vi "Update Plugin Status.vi"(6 "channels":T1, 8 "error in (no error)":errorcluster, 9 "Status":T5, 10 "Plugin Name":string, 11 "Launcher in":refnum<class "CIFPluginManager.lvclass">) -> (0 "error out":errorcluster)   [LabVIEW 2021, in "CIFPluginManager.lvclass"]
uses:
  CIFPluginManager.lvclass
  CIFPluginManager.lvclass/CIFPluginManager.ctl
  <vilib>/Utility/miscctls.llb/LVMapReplaceAction.ctl
  gRPC/CIF_Manager_server/RPC Messages/cif_management_common_PluginStatusData.ctl
  gRPC/CIF_Manager_server/CIF_Manager_server.lvlib
  gRPC/CIF_Manager_server/RPC Messages/cif_common_TimingStats.ctl
  gRPC/CIF_Manager_server/RPC Messages/cif_management_common_Channels.ctl
  gRPC/CIF_Manager_server/RPC Messages/cif_management_common_MonitorI64.ctl
  gRPC/CIF_Manager_server/RPC Messages/cif_management_common_MonitorU64.ctl
  gRPC/CIF_Manager_server/RPC Messages/cif_management_common_MonitorDoubles.ctl
  gRPC/CIF_Manager_server/RPC Messages/cif_management_common_Error.ctl
  gRPC/CIF_Manager_server/RPC Messages/cif_management_common_FifoStatistics.ctl
  gRPC/CIF_Manager_server/RPC Messages/cif_management_common_TimingStatistics.ctl
  gRPC/CIF_Manager_server/RPC Messages/cif_management_common_PluginStatusData_PluginState.ctl
  gRPC/CIF_Manager_server/RPC Messages/cif_management_common_ChannelPattern.ctl
  gRPC/CIF_Manager_server/RPC Messages/cif_management_common_ChannelDirection.ctl
  gRPC/CIF_Manager_server/RPC Messages/cif_management_common_Channel.ctl
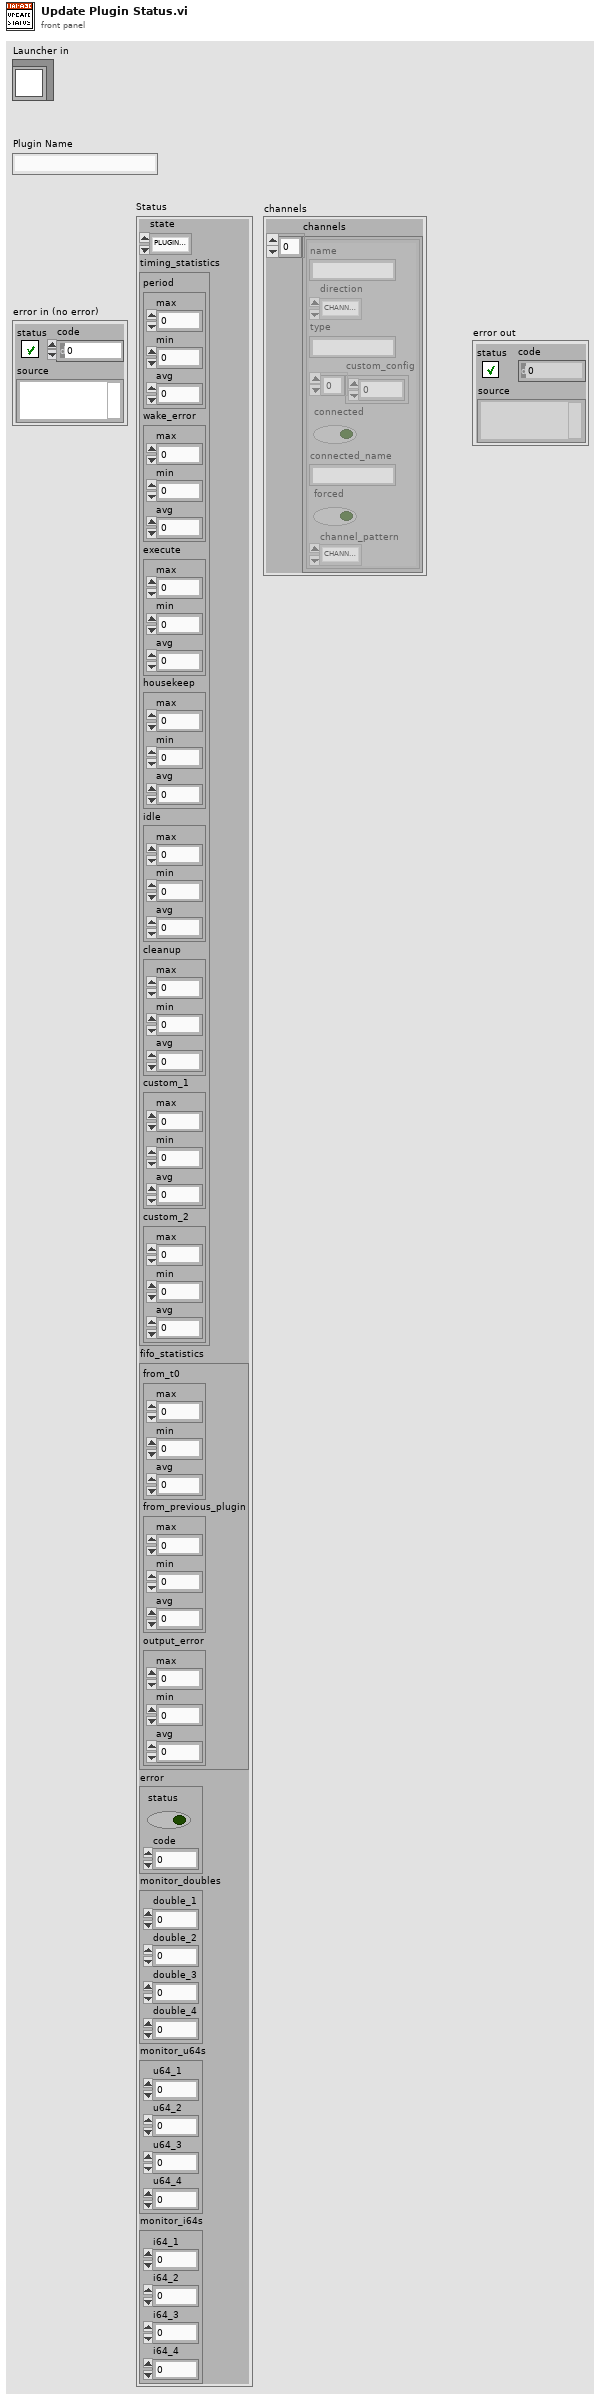
[diagram p1: front panel]
types:
  T1 = typedef "CIF_Manager_server.lvlib/cif_management_common_Channels.ctl" = cluster{"channels":T2[]}
  T2 = typedef "CIF_Manager_server.lvlib/cif_management_common_Channel.ctl" = cluster{"name":string, "direction":T3, "type":string, "custom_config":u8[], "connected":bool, "connected_name":string, "forced":bool, "channel_pattern":T4}
  T3 = typedef "CIF_Manager_server.lvlib/cif_management_common_ChannelDirection.ctl" = enum32{"CHANNELDIRECTION_UNKNOWN", "CHANNELDIRECTION_PUBLISHER", "CHANNELDIRECTION_SUBSCRIBER"}
  T4 = typedef "CIF_Manager_server.lvlib/cif_management_common_ChannelPattern.ctl" = enum32{"CHANNELPATTERN_UNKNOWN", "CHANNELPATTERN_TAG", "CHANNELPATTERN_FIFO", "CHANNELPATTERN_MULTIFIFO", "CHANNELPATTERN_BACKPRESSUREFIFO"}
  T5 = typedef "CIF_Manager_server.lvlib/cif_management_common_PluginStatusData.ctl" = cluster{"state":T6, "timing_statistics":T7, "fifo_statistics":T9, "error":T10, "monitor_doubles":T11, "monitor_u64s":T12, "monitor_i64s":T13}
  T6 = typedef "CIF_Manager_server.lvlib/cif_management_common_PluginStatusData_PluginState.ctl" = enum32{"PLUGINSTATE_UNKNOWN", "PLUGINSTATE_CREATING", "PLUGINSTATE_LISTENING", "PLUGINSTATE_RUNNING", "PLUGINSTATE_CLEANINGUP", "PLUGINSTATE_DESTROYING"}
  T7 = typedef "CIF_Manager_server.lvlib/cif_management_common_TimingStatistics.ctl" = cluster{"period":T8, "wake_error":T8, "execute":T8, "housekeep":T8, "idle":T8, "cleanup":T8, "custom_1":T8, "custom_2":T8}
  T8 = typedef "CIF_Manager_server.lvlib/cif_common_TimingStats.ctl" = cluster{"max":i64, "min":i64, "avg":dbl}
  T9 = typedef "CIF_Manager_server.lvlib/cif_management_common_FifoStatistics.ctl" = cluster{"from_t0":T8, "from_previous_plugin":T8, "output_error":T8}
  T10 = typedef "CIF_Manager_server.lvlib/cif_management_common_Error.ctl" = cluster{"status":bool, "code":i32}
  T11 = typedef "CIF_Manager_server.lvlib/cif_management_common_MonitorDoubles.ctl" = cluster{"double_1":dbl, "double_2":dbl, "double_3":dbl, "double_4":dbl}
  T12 = typedef "CIF_Manager_server.lvlib/cif_management_common_MonitorU64.ctl" = cluster{"u64_1":u64, "u64_2":u64, "u64_3":u64, "u64_4":u64}
  T13 = typedef "CIF_Manager_server.lvlib/cif_management_common_MonitorI64.ctl" = cluster{"i64_1":i64, "i64_2":i64, "i64_3":i64, "i64_4":i64}
  T14 = typedef "LVMapReplaceAction.ctl" = enum32{"Modify Entry only if found", "Add or Modify Entry", "Delete Entry"}
  T15 = typedef "CIFPluginManager.lvclass/Plugin Management Data Map.ctl" = map{string, T16}
  T16 = typedef "CIFPluginManager.lvclass/Plugin Management Data.ctl" = cluster{"Unique Name":string, "Plugin Type":string, "gRPC Port":i32, "gRPC ID":T17, "Loader Type":T18, "Loader":string, "Version":T19, "Load Timestamp":i64, "Unload Timestamp":i64, "Unloading":bool, "Ready for removal":bool, "status":T5, "channels":T1}
  T17 = typedef "grpc-lvsupport-release.lvlib/grpcId.ctl" = u64
  T18 = typedef "CIFPluginManager.lvclass/Loader Type.ctl" = enum16{"LabVIEW"}
  T19 = typedef "CIFCoreCommon.lvlib/Version.ctl" = cluster{"Major":i32, "Minor":i32, "Fix":i32, "Build":i32}
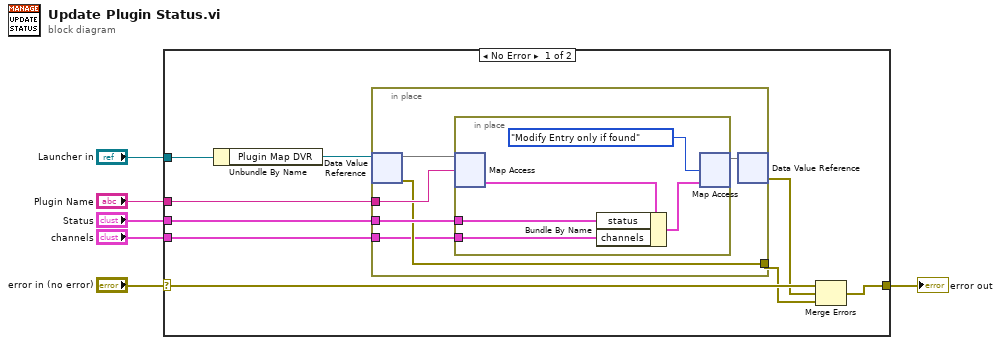
[diagram p0: block diagram]
diagram:
  n1 = case shown="No Error" "error in (no error)" {
    selector: "error in (no error)" -> [w11 w27]
    tunnel: [w8 w27] -> w5
    tunnel: "Launcher in" -> [w13 _]
    tunnel: "Plugin Name" -> [w15 _]
    tunnel: "Status" -> [w14 _]
    tunnel: "channels" -> [w7 _]
    frame No Error {
      n2 = Unbundle By Name(w13) -> ("Plugin Map DVR"=w12:refnum<data-value>)
      n3 = in-place {
        in-place-border: w15 -> [w21]
        in-place-border: w14 -> [w20]
        in-place-border: [w18] -> w9
        in-place-border: w7 -> [w16]
        n4 = in-place-dvr #1(w12) -> (w19:T15, w18:errorcluster)
        n5 = in-place {
          in-place-border: w20 -> [w24]
          in-place-border: w16 -> [w22]
          n6 = in-place-map #2(w19, w21) -> (w25:T16)  [unwired: 1 in, 1 out]
          n7 = Bundle By Name(cluster=w25, "status"=w24, "channels"=w22) -> (w23:T16)
          n8 = in-place-map #2(w23, LVMapReplaceAction."Modify Entry only if found" ("action")) -> (w17:T15)  [unwired: 2 out]
        }
        n9 = in-place-dvr #1(w17) -> (w10:errorcluster)  [unwired: 1 out]
      }
      n10 = Merge Errors(w11, w10, w9) -> (w8:errorcluster)
    }
    frame Error {
    }
  }
  "error out" <- w5
